vi "主程序-生产消费.vi"() -> ()   [LabVIEW 2013]
doc: "该模板用于创建生产者／消费者模式的应用程序，以事件驱动的方式，生成队列中的项。如需通过响应事件实现代码的异步执行，同时不影响用户界面的响应速度，可考虑用该模式替代“用户界面事件处理器”模式。"
uses:
  <vilib>/Instr/_visa.llb/VISA Configure Serial Port (Instr).vi
panel:
  out "CRC校验位":string
  out "运行速度（256-65535）":i32
  in  "减速（Max=65535）":i32=550
  in  "加速（Max=65535）":i32=550
  in  "位置控制模式":bool=TRUE
  in  "行进距离（Max=16777214）":i32
  out "验证":string
  out "abc":string
  in  "执行次数":i32=3
  in  "模式选择":string(combo)="\u0000"
  out "低位":string
  out "高位":string
  in  "速度增减幅度":u16(ring)=1 items=["1"=1, "10"=10, "20"=20, "50"=50, "100"=100, "200"=200, "500"=500, "1000"=1000, "2000"=2000, "5000"=5000, "10000"=10000]
  in  "速度-":bool
  in  "速度+":bool
  in  "运行速度":i32=63500
  in  "停止运行":bool
  in  "负向运行":bool
  in  "正向运行":bool
  in  "停止":bool
  in  "端口开关":bool
  in  "端口选择":refnum<visa-resource-name>
  # "步进电机控制系统"
  # "请关闭端口开关后再停止程序！"
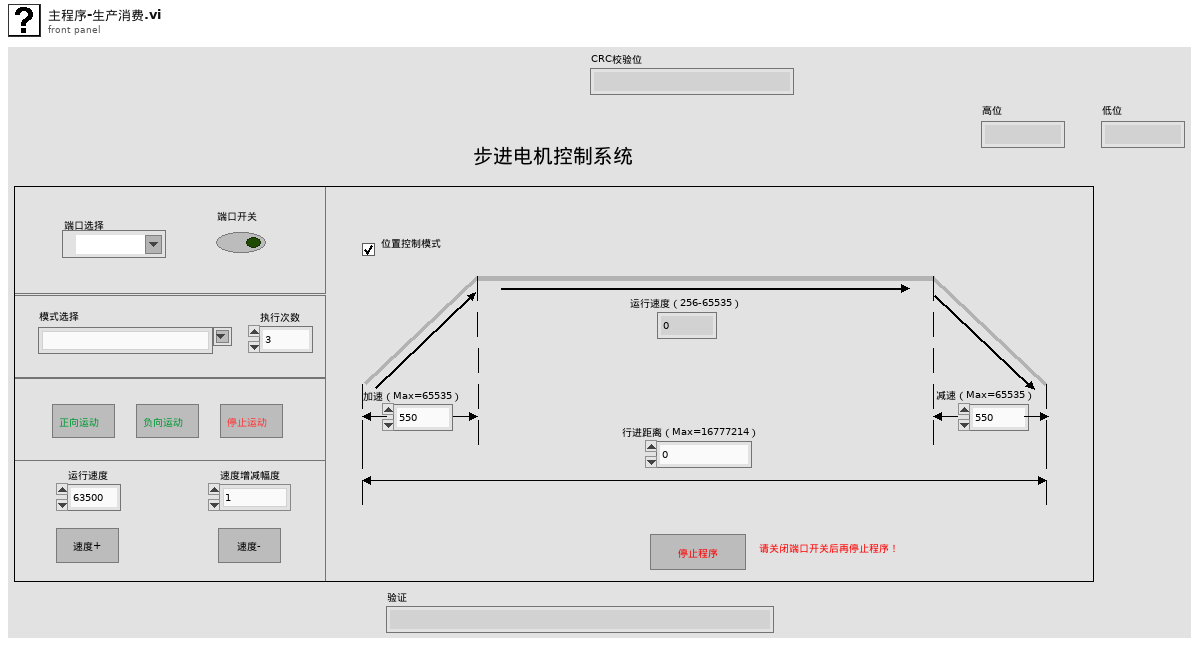
[diagram p1: front panel]
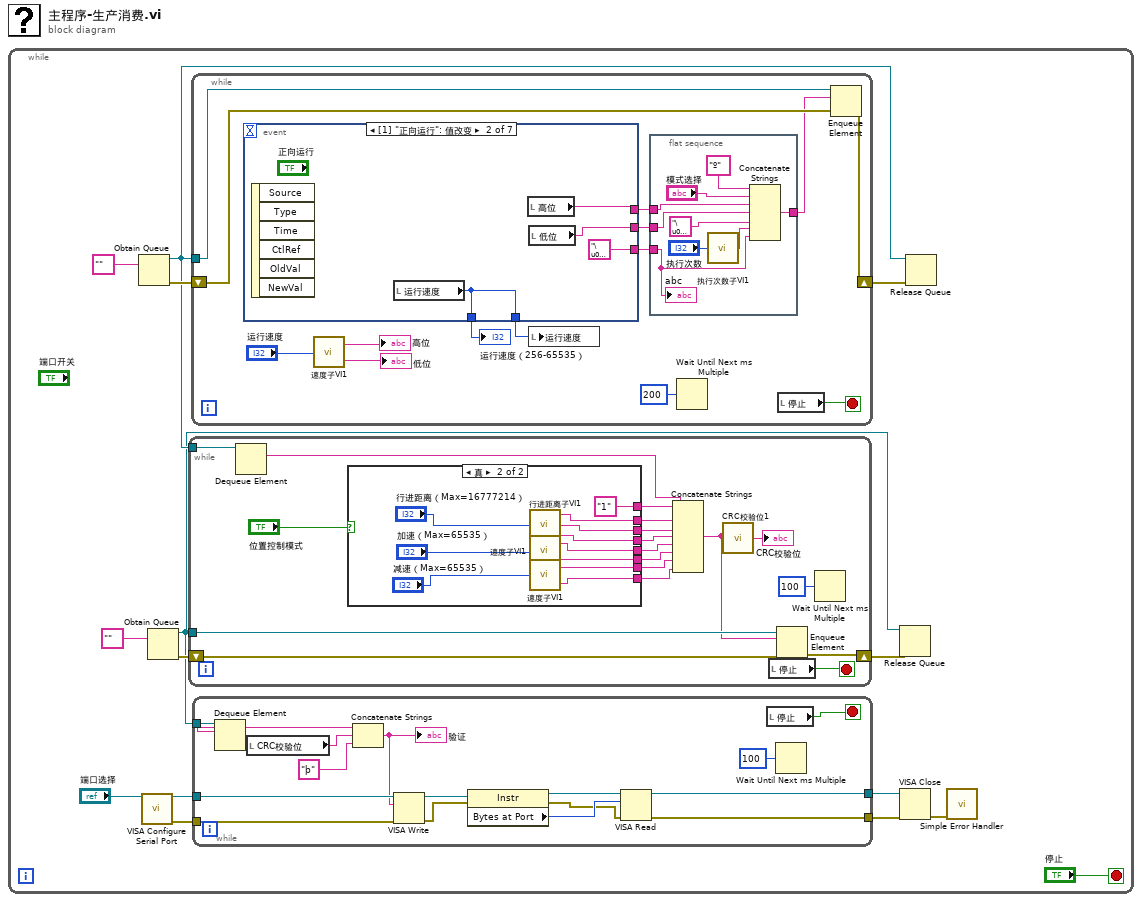
[diagram p0: block diagram]
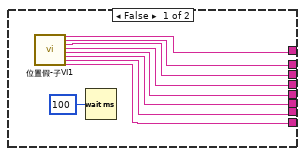
[diagram p2: hidden frame]
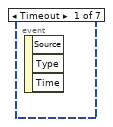
[diagram p3: hidden frame]
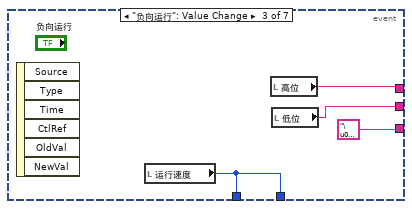
[diagram p4: hidden frame]
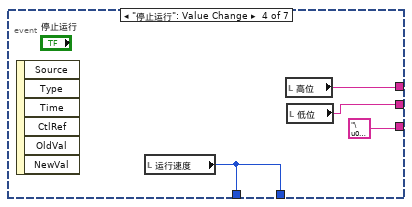
[diagram p5: hidden frame]
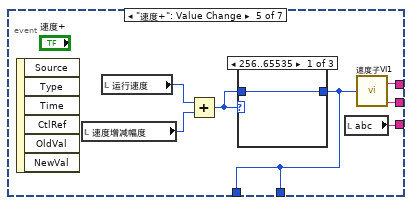
[diagram p6: hidden frame]
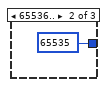
[diagram p7: hidden frame]
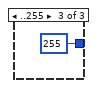
[diagram p8: hidden frame]
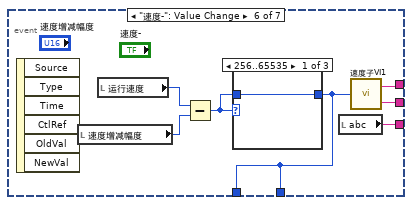
[diagram p9: hidden frame]
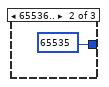
[diagram p10: hidden frame]
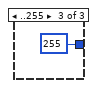
[diagram p11: hidden frame]
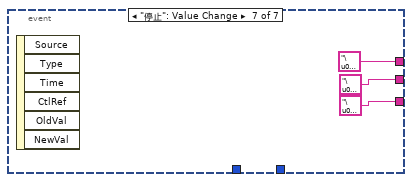
[diagram p12: hidden frame]
diagram:
  n1 = while {
    stop <- "停止" stop-if-true
    n2 = Obtain Queue(element data type="") -> (queue out=w6:refnum<queue>, error out=w15:errorcluster)  [unwired: 4 in, 1 out]
    n3 = call-poly "VISA Configure Serial Port"("VISA resource name"="端口选择") -> ("VISA resource name out"=w12:refnum<visa-resource-name>, "error out"=w11:errorcluster)  [unwired: 13 in]
    n4 = Obtain Queue(element data type="") -> (queue out=w2:refnum<queue>, error out=w4:errorcluster)  [unwired: 4 in, 1 out]
    n5 = while {
      tunnel: w6 -> [w25]
      tunnel: w2 -> [w23]
      shift-right: [w21] -> w3
      shift-left: w4 -> [w22]
      stop <- w18 stop-if-true
      n6 = Dequeue Element(queue=w25) -> (element=w24:string)  [unwired: 2 in, 3 out]
      n7 = case shown="真" "位置控制模式" {
        tunnel: [w35 w53] -> w33
        tunnel: [w36 w52] -> w32
        tunnel: [w37 w51] -> w31
        tunnel: [w38 w50] -> w30
        tunnel: [w39 w49] -> w29
        tunnel: [w40 w48] -> w28
        tunnel: [w41 w47] -> w27
        tunnel: [w42 "1"] -> w26
        frame False {
          n8 = call "位置假-子VI1.vi"() -> ("8"=w42:string, "9"=w41:string, "10"=w40:string, "11"=w39:string, "12"=w38:string, "13"=w37:string, "14"=w36:string, "15"=w35:string)  [unwired: 20 in]
          n9 = Wait (ms)(milliseconds to wait=u32 100 ("等待时间（毫秒）")) -> ()  [unwired: 1 out]
        }
        frame True {
          n10 = call "行进距离子VI1.vi"("脉冲输入端"="行进距离（Max=16777214）") -> ("行进脉冲总数高位"=w47:string, "行进脉冲总数中位"=w48:string, "行进脉冲总数低位"=w49:string)
          n11 = call "速度子VI1.vi"("脉冲数"="加速（Max=65535）") -> ("分频基数高位"=w50:string, "分频基数低位"=w51:string)
          n12 = call "速度子VI1.vi"("脉冲数"="减速（Max=65535）") -> ("分频基数高位"=w52:string, "分频基数低位"=w53:string)
        }
      }
      n13 = Concatenate Strings(w24, w26, w27, w28, w29, w30, w31, w32, w33) -> (w19:string)
      n14 = call "CRC校验位1.vi"("输入端"=w19) -> ("CRC校验位"=→"CRC校验位":string)
      n15 = local read "停止"() -> (w18:bool)
      n16 = Enqueue Element(queue=w23, element=w19, error in (no error)=w22) -> (error out=w21:errorcluster)  [unwired: 1 in, 2 out]
      n17 = Wait Until Next ms Multiple(millisecond multiple=u32 100 ("毫秒倍数")) -> ()  [unwired: 1 out]
    }
    n18 = while {
      shift-right: [w78] -> w14
      shift-left: w15 -> [w83]
      tunnel: w6 -> [w82]
      stop <- w71 stop-if-true
      n19 = event shown="[1] \"正向运行\": 值改变" {
        selector: _ -> [_ _ _ _ _ _ _]
        dyn-events: _ -> [_ _ _ _ _ _ _]
        timeout: _ -> [_ _ _ _ _ _ _]
        tunnel: [_ w96 w100 w104 w108 w118 "\u0000"] -> w75
        tunnel: [_ w95 w99 w103 w107 w117 "\u0000"] -> w74
        tunnel: [_ "\u0001" "\u0002" "\u0003" w106 w116 "\u0000"] -> w73
        tunnel: [_ w93 w97 w101 w105 w115 _] -> w77
        tunnel: [_ w93 w97 w101 w105 w115 _] -> w76
        event Timeout {
          n20 = event-data() -> ()  [unwired: 1 in, 3 out]
        }
        event "正向运行": Value Change {
          n21 = event-data() -> ()  [unwired: 1 in, 6 out]
          n22 = local read "运行速度"() -> (w93:i32)
          n23 = local read "高位"() -> (w96:string)
          n24 = local read "低位"() -> (w95:string)
        }
        event "负向运行": Value Change {
          n25 = event-data() -> ()  [unwired: 1 in, 6 out]
          n26 = local read "运行速度"() -> (w97:i32)
          n27 = local read "高位"() -> (w100:string)
          n28 = local read "低位"() -> (w99:string)
        }
        event "停止运行": Value Change {
          n29 = event-data() -> ()  [unwired: 1 in, 6 out]
          n30 = local read "运行速度"() -> (w101:i32)
          n31 = local read "高位"() -> (w104:string)
          n32 = local read "低位"() -> (w103:string)
        }
        event "速度+": Value Change {
          n33 = event-data() -> ()  [unwired: 1 in, 6 out]
          n34 = local read "速度增减幅度"() -> (w110:u16)
          n35 = local read "运行速度"() -> (w111:i32)
          n36 = Add(x=w111, y=w110) -> (x+y=w109:i32)
          n37 = case shown="256..65535" w109 {
            tunnel: w109 -> [w112 _ _]
            tunnel: [w112 65535 255] -> w105
            frame 256..65535 {
            }
            frame 65536.. {
            }
            frame ..255 {
            }
          }
          n38 = local read "abc"() -> (w106:string)
          n39 = call "速度子VI1.vi"("脉冲数"=w105) -> ("分频基数高位"=w108:string, "分频基数低位"=w107:string)
        }
        event "速度-": Value Change {
          n40 = event-data() -> ()  [unwired: 1 in, 6 out]
          n41 = local read "速度增减幅度"() -> (w120:u16)
          n42 = local read "运行速度"() -> (w121:i32)
          n43 = Subtract(x=w121, y=w120) -> (x-y=w119:i32)
          n44 = case shown="256..65535" w119 {
            tunnel: w119 -> [w122 _ _]
            tunnel: [w122 65535 255] -> w115
            frame 256..65535 {
            }
            frame 65536.. {
            }
            frame ..255 {
            }
          }
          n45 = local read "abc"() -> (w116:string)
          n46 = call "速度子VI1.vi"("脉冲数"=w115) -> ("分频基数高位"=w118:string, "分频基数低位"=w117:string)
        }
        event "停止": Value Change {
          n47 = event-data() -> ()  [unwired: 1 in, 6 out]
        }
      }
      "运行速度（256-65535）" <- w77
      n48 = call "速度子VI1.vi"("脉冲数"="运行速度") -> ("分频基数高位"=→"高位":string, "分频基数低位"=→"低位":string)
      n49 = local write "运行速度"(w76) -> ()
      n50 = flat-sequence {
        tunnel: w75 -> [w90]
        tunnel: w74 -> [w89]
        tunnel: w73 -> [w86]
        tunnel: [w84] -> w72
        frame #0 {
          n51 = call "执行次数子VI1.vi"("执行次数"="执行次数") -> ("HEX显示"=w87:string)
          n52 = Concatenate Strings("º" ("字符串"), "模式选择", w90, w89, "\u0000", w87, w86) -> (w84:string)
          "abc" <- w86
        }
      }
      n53 = Wait Until Next ms Multiple(millisecond multiple=u32 200 ("毫秒倍数")) -> ()  [unwired: 1 out]
      n54 = local read "停止"() -> (w71:bool)
      n55 = Enqueue Element(queue=w82, element=w72, error in (no error)=w83) -> (error out=w78:errorcluster)  [unwired: 1 in, 2 out]
    }
    n56 = while {
      tunnel: w12 -> [w69]
      tunnel: w11 -> [w68]
      tunnel: [w62] -> w8
      tunnel: [w61] -> w7
      tunnel: w2 -> [w60]
      stop <- w56 stop-if-true
      n57 = Dequeue Element(queue=w60) -> (element=w59:string)  [unwired: 2 in, 3 out]
      n58 = local read "CRC校验位"() -> (w58:string)
      n59 = Concatenate Strings(w59, w58, "þ" ("字符串")) -> (w55:string)
      "验证" <- w55
      n60 = VISA Write(VISA resource name=w69, write buffer=w55, error in (no error)=w68) -> (VISA resource name out=w67:refnum<visa-resource-name>, error out=w66:errorcluster)  [unwired: 1 out]
      n61 = property class="Instr"(reference=w67, error in=w66) -> (reference out=w63:refnum<visa-resource-name>, error out=w64:errorcluster, "Bytes at Port"=w65:u32)
      n62 = VISA Read(VISA resource name=w63, byte count=w65, error in (no error)=w64) -> (VISA resource name out=w62:refnum<visa-resource-name>, error out=w61:errorcluster)  [unwired: 2 out]
      n63 = local read "停止"() -> (w56:bool)
      n64 = Wait Until Next ms Multiple(millisecond multiple=u32 100 ("毫秒倍数")) -> ()  [unwired: 1 out]
    }
    n65 = Release Queue(queue=w2, error in (no error)=w3) -> ()  [unwired: 1 in, 3 out]
    n66 = VISA Close(VISA resource name=w8, error in (no error)=w7) -> (error out=w9:errorcluster)
    n67 = Release Queue(queue=w6, error in (no error)=w14) -> ()  [unwired: 1 in, 3 out]
    n68 = call <vilib>:"Simple Error Handler.vi"("error in (no error)"=w9) -> ()  [unwired: 4 in, 5 out]
  }
